vi "PH_Synchrolock_Watch.PC Write PSDB.vi"(0 "i ref in":refnum<vi>, 5 "error IO":errorcluster) -> (14 "i ref out":refnum<vi>, 19 "error out":errorcluster)   [LabVIEW 2014, in "PH_Synchrolock_Watch.lvlib"]
doc: "This is the proc case which writes data to the PHELIX shot data base."
uses:
  PH_Synchrolock_Watch.lvlib
  PH_StatusHandler/PH_StatusHandler.lvlib
  PH_TKTDS-30xx/PH_TKTDS-30xx.lvlib
  PH_PSDBWriter/PH_PSDBWriter.lvlib
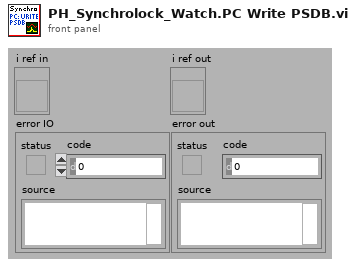
[diagram p1: front panel]
types:
  T1 = typedef "PH_TKTDS-30xx.lvlib/PH_TKTDS-30xx.i attribute.ctl" = cluster{"Default VISA Resource":string, "VISA Resource Name":refnum<visa-resource-name>, "Revision":cluster{"Instrument Driver":string, "Instrument Firmware":string}, "Selftest":cluster{"Result":u32, "Message":string}, "Channels":T2[], "Trigger Configuration":T3, "Acquisition Configuration":T4, "Fetched Waveforms":T5[], "GUI Refs":T6, "GUI Refs Channels":refnum<vi>[], "State":T7, "Error Message":string, "Allow Prdc Loop?":bool}
  T2 = typedef "PH_TKTDS-30xx.lvlib/PH_TKTDS-30xx.Channel Config.ctl" = cluster{"Channel Name":string, "Input Impedance":string, "Max Input Frequency":string, "Vertical Coupling":i32, "Channel Enabled":bool, "Probe Attenuation":dbl, "Vertical Range":dbl, "Vertical Offset":dbl}
  T3 = typedef "PH_TKTDS-30xx.lvlib/PH_TKTDS-30xx.Trigger Config.ctl" = cluster{"Source":string, "Slope":i32, "Level [V]":dbl}
  T4 = typedef "PH_TKTDS-30xx.lvlib/PH_TKTDS-30xx.Acquisition Config.ctl" = cluster{"Time base":dbl, "Record Length":u16, "Start Time":dbl, "Type":i32, "Continuous":bool}
  T5 = typedef "PH_TKTDS-30xx.lvlib/PH_TKTDS-30xx.fetched Waveform.ctl" = cluster{"Source":string, "Actual Points":u32, "Initial X":dbl, "X Increment":dbl, "Waveform Array":dbl[]}
  T6 = typedef "PH_TKTDS-30xx.lvlib/PH_TKTDS-30xx.GUI Refs.ctl" = cluster{"Trigger":refnum<vi>, "Acquisition":refnum<vi>, "Graph":refnum<vi>, "State":refnum<vi>, "Delete":refnum<vi>, "Channel to be positioned":refnum<vi>, "Postion":refnum<vi>, "Display Intensity":refnum<vi>, "VISA Resource":refnum<vi>}
  T7 = typedef "PH_StatusHandler.lvlib/PH_StatusHandler.Status.ctl" = i16
  T8 = typedef "PH_PSDBWriter.lvlib/PH_PSDBWriter.Boolean dataset.ctl" = cluster{"name":string, "data":bool, "unit":string}
  T9 = typedef "PH_PSDBWriter.lvlib/PH_PSDBWriter.String dataset.ctl" = cluster{"name":string, "data":string, "unit":string}
  T10 = typedef "PH_PSDBWriter.lvlib/PH_PSDBWriter.PSDB Dataset.ctl" = cluster{"Version":i32, "2D data Input":T11[], "Boolean Input":T8[], "Image Input":T13[], "Numeric Input":T15[], "String Input":T9[]}
  T11 = typedef "PH_PSDBWriter.lvlib/PH_PSDBWriter.2D dataset.ctl" = cluster{"name":string, "data":dbl[][], "axis description":T12}
  T12 = typedef "PSDB.lvlib/PSDB_AxisDescription.ctl" = cluster{"x axis label":string, "y axis label":string, "x axis unit":string, "y axis unit":string}
  T13 = typedef "PH_PSDBWriter.lvlib/PH_PSDBWriter.Image dataset.ctl" = cluster{"name":string, "data":T14, "unit":string}
  T14 = typedef "IMAQ Image.ctl" = refnum<image>
  T15 = typedef "PH_PSDBWriter.lvlib/PH_PSDBWriter.Numeric dataset.ctl" = cluster{"name":string, "data":dbl, "unit":string}
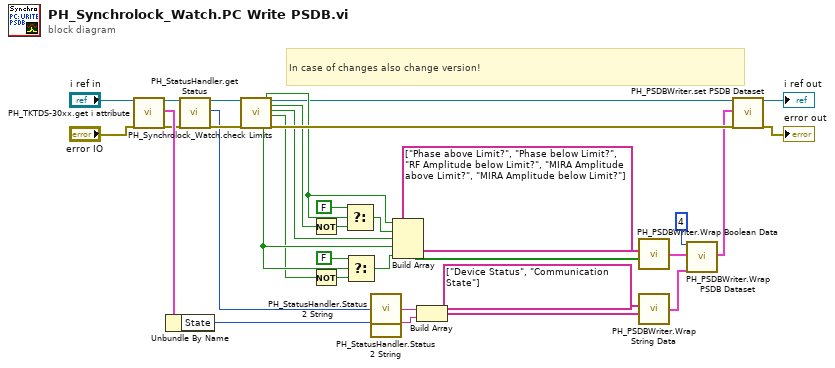
[diagram p0: block diagram]
diagram:
  # "In case of changes also change version!"
  n1 = call "PH_TKTDS-30xx.get i attribute.vi"("i ref in"="i ref in", "error in (no error)"="error IO") -> ("i ref out"=w33:refnum<vi>, "i attribute"=w34:T1, "error out"=w32:errorcluster)  [unwired: 15 in]
  n2 = Unbundle By Name(w34) -> ("State"=w28:T7)
  n3 = call "PH_StatusHandler.get Status.vi"("VI in"=w33, "error in"=w32) -> ("VI out"=w24:refnum<vi>, "Status"=w1:T7, "error out"=w29:errorcluster)  [unwired: 15 in]
  n4 = call "PH_Synchrolock_Watch.check Limits.vi"("i ref in"=w24, "error in"=w29) -> ("Phase above Limit?"=w13:bool, "MIRA above Limit?"=w17:bool, "i ref out"=w11:refnum<vi>, "Phase in range?"=w20:bool, "RF Amplitude below Limit?"=w23:bool, "MIRA Amplitude in range?"=w15:bool, "error out"=w25:errorcluster)  [unwired: 11 in]
  n5 = Not(x=w20) -> (.not. x?=w19:bool)
  n6 = Not(x=w15) -> (.not. x?=w16:bool)
  n7 = Select(t=FALSE, s=w13, f=w19) -> (s? t:f=w21:bool)
  n8 = Select(t=FALSE, s=w17, f=w16) -> (s? t:f=w14:bool)
  n9 = call "PH_StatusHandler.Status 2 String.vi"("Status"=w1) -> ("Status as string"=w26:string)
  n10 = call "PH_StatusHandler.Status 2 String.vi"("Status"=w28) -> ("Status as string"=w27:string)
  n11 = Build Array(w13, w21, w23, w17, w14) -> (w5:bool[])
  n12 = Build Array(w26, w27) -> (w2:string[])
  n13 = call "PH_PSDBWriter.Wrap Boolean Data.vi"("Data Array"=w5, "Name Array"=string[] ["Phase above Limit?", "Phase below Limit?", "RF Amplitude below Limit?", "MIRA Amplitude above Limit?", "MIRA Amplitude below Limit?"]) -> ("PSDB Boolean Data Array"=w7:T8[])  [unwired: 2 in]
  n14 = call "PH_PSDBWriter.Wrap String Data.vi"("Data Array"=w2, "Name Array"=string[] ["Device Status", "Communication State"]) -> ("PSDB String Data Array"=w4:T9[])  [unwired: 2 in]
  n15 = call "PH_PSDBWriter.Wrap PSDB Dataset.vi"("Version"=4, "Boolean Input"=w7, "String Input"=w4) -> ("PSDB Dataset"=w9:T10)  [unwired: 16 in]
  n16 = call "PH_PSDBWriter.set PSDB Dataset.vi"("VI in"=w11, "PSDB Dataset"=w9, "error in (no error)"=w25) -> ("VI out"=→"i ref out":refnum<vi>, "error out"=→"error out":errorcluster)  [unwired: 15 in]
